vi "setpoints.vi"() -> ()   [LabVIEW 2013]
uses:
  <vilib>/Utility/file.llb/Read From Spreadsheet File (DBL).vi
  Robot Global Data.vi
panel:
  in  "Default File":i32
  out "Number of Auton Files":i64
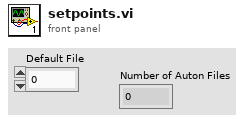
[diagram p1: front panel]
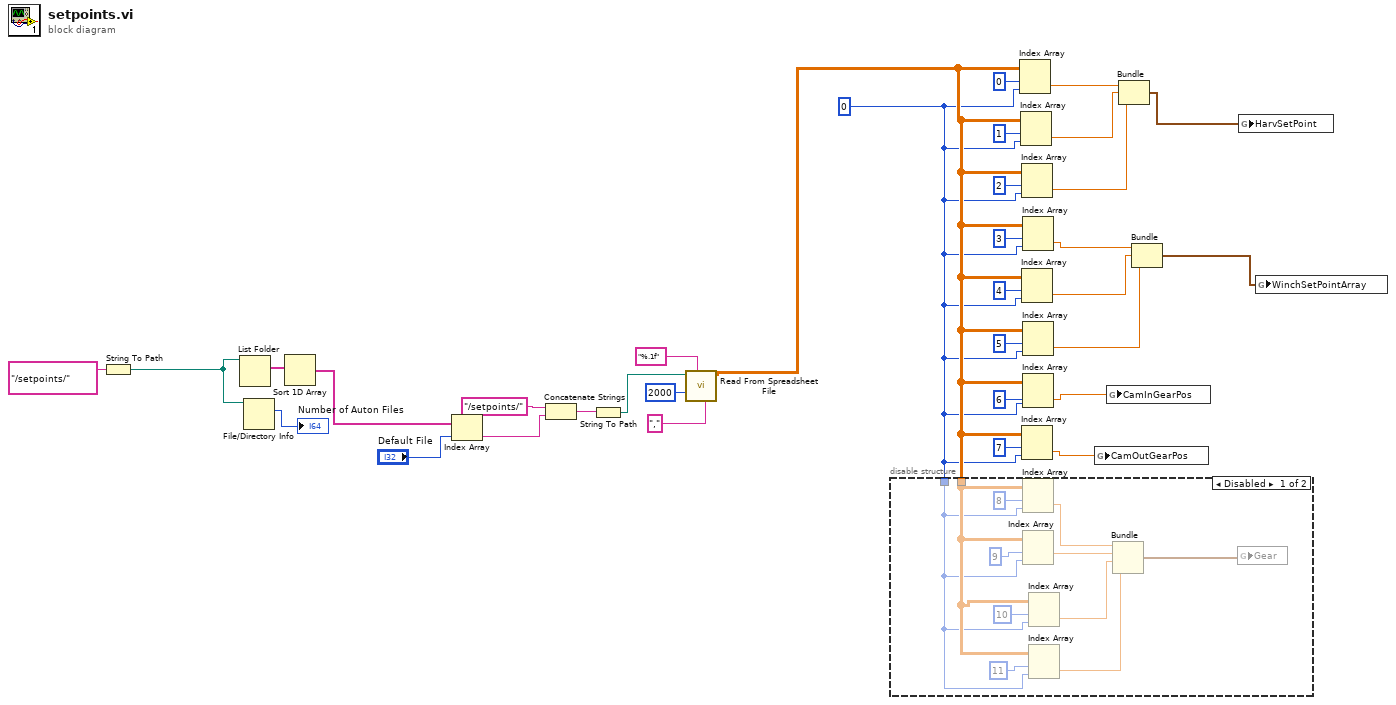
[diagram p0: block diagram]
diagram:
  w1 = 0
  n1 = String To Path(string="/setpoints/") -> (path=w24:path)
  n2 = List Folder(path=w24) -> (filenames=w25:string[])  [unwired: 1 in, 5 out]
  n3 = File/Directory Info(path=w24) -> (size=→"Number of Auton Files":i64)  [unwired: 1 in, 6 out]
  n4 = Sort 1D Array(array=w25) -> (sorted array=w27:string[])
  n5 = Index Array(array=w27, index="Default File") -> (element=w22:string)
  n6 = Concatenate Strings("/setpoints/" ("string"), w22) -> (w30:string)
  n7 = String To Path(string=w30) -> (path=w29:path)
  n8 = call-poly <vilib>:"Read From Spreadsheet File.vi"("delimiter (\\t)"="," ("delimiter (\\t)"), "format (%.3f)"="%.1f", "number of rows (all:-1)"=2000, "file path (dialog if empty)"=w29) -> ("all rows"=w2:dbl[][])  [unwired: 1 in, 6 out]
  n9 = disable-structure shown="Disabled" {
    disable-tunnel: w2 -> [w40 _]
    disable-tunnel: w1 -> [w39 _]
    frame Disabled {
      n10 = Index Array(array=w40, index (row)=8, index (col)=w39) -> (element=w38:dbl)
      n11 = Index Array(array=w40, index (row)=9, index (col)=w39) -> (element=w37:dbl)
      n12 = Index Array(array=w40, index (row)=10, index (col)=w39) -> (element=w36:dbl)
      n13 = Index Array(array=w40, index (row)=11, index (col)=w39) -> (element=w35:dbl)
      n14 = Bundle(w38, w37, w36, w35) -> (w34:cluster{dbl, dbl, dbl, dbl})  [unwired: 1 in]
      n15 = global write "Robot Global Data.vi" "Gear"(w34) -> ()
    }
    frame Enabled {
    }
  }
  n16 = Index Array(array=w2, index (row)=0, index (col)=w1) -> (element=w12:dbl)
  n17 = Index Array(array=w2, index (row)=1, index (col)=w1) -> (element=w11:dbl)
  n18 = Index Array(array=w2, index (row)=2, index (col)=w1) -> (element=w10:dbl)
  n19 = Index Array(array=w2, index (row)=4, index (col)=w1) -> (element=w7:dbl)
  n20 = Index Array(array=w2, index (row)=7, index (col)=w1) -> (element=w4:dbl)
  n21 = Index Array(array=w2, index (row)=3, index (col)=w1) -> (element=w8:dbl)
  n22 = Index Array(array=w2, index (row)=5, index (col)=w1) -> (element=w6:dbl)
  n23 = Index Array(array=w2, index (row)=6, index (col)=w1) -> (element=w3:dbl)
  n24 = global write "Robot Global Data.vi" "CamOutGearPos"(w4) -> ()
  n25 = global write "Robot Global Data.vi" "CamInGearPos"(w3) -> ()
  n26 = Bundle(w12, w11, w10) -> (w9:cluster{dbl, dbl, dbl})  [unwired: 1 in]
  n27 = Bundle(w8, w7, w6) -> (w5:cluster{dbl, dbl, dbl})  [unwired: 1 in]
  n28 = global write "Robot Global Data.vi" "HarvSetPoint"(w9) -> ()
  n29 = global write "Robot Global Data.vi" "WinchSetPointArray"(w5) -> ()
